vi "SLL DE DAQ Parameters LV2 Global.vi"(6 "Option":T6, 8 "Error in (no error)":errorcluster, 11 "Global Info":T1={"Enable Engines"={"AI Enable"=TRUE, "AO Enable"=TRUE, "DI Enable"=TRUE, "DO Enable"=TRUE}, "DAQ Control Type"={"Analog Input"=enum."Finite", "Analog Output"=enum."Finite", "Digital Input"=enum."Finite", "Digital Output"=enum."Finite"}, "DAQ Parameters"={"AI Sampling Rate (Samples/Sec)"=1000.0, "MvgAVG Window Size (# of Points)"=1000, "Enable Filter"=TRUE, "Enable MvgAVG"=TRUE, "Circular Buffer Size (Sec)"=1000.0, "AO Sampling Rate (Samples/Sec)"=1000.0, "Graph Update Rate (Samples/Sec)"=0.0, "File Logging Rate (Samples/Sec)"=500}, "AO Safe Values"=[], "DO Safe Values"=[], "DO Interconnected Lines"=[], "AI Channels Unit"=[], "Units Information"=[]}) -> (0 "Error out":errorcluster, 3 "Global Info":T1={"Enable Engines"={"AI Enable"=TRUE, "AO Enable"=TRUE, "DI Enable"=TRUE, "DO Enable"=TRUE}, "DAQ Control Type"={"Analog Input"=enum."Finite", "Analog Output"=enum."Finite", "Digital Input"=enum."Finite", "Digital Output"=enum."Finite"}, "DAQ Parameters"={"AI Sampling Rate (Samples/Sec)"=1000.0, "MvgAVG Window Size (# of Points)"=1000, "Enable Filter"=TRUE, "Enable MvgAVG"=TRUE, "Circular Buffer Size (Sec)"=1000.0, "AO Sampling Rate (Samples/Sec)"=1000.0, "Graph Update Rate (Samples/Sec)"=0.0, "File Logging Rate (Samples/Sec)"=500}, "AO Safe Values"=[], "DO Safe Values"=[], "DO Interconnected Lines"=[], "AI Channels Unit"=[], "Units Information"=[]})   [LabVIEW 2013]
uses:
  Sub VIs/DAQ Engine/Controls/SLL DE DAQ Parameters LV2Global Options.ctl
  Sub VIs/DAQ Engine/Controls/SLL DE DAQ Engine Parameters.ctl
  Sub VIs/DAQ Engine/Controls/SLL DE List of Analog Outputs.ctl
  Sub VIs/DAQ Engine/Controls/SLL DE List of Digital Outputs.ctl
  Sub VIs/DAQ Engine/Controls/SLL DE List of Analog Inputs.ctl
  Sub VIs/DAQ Engine/Controls/SLL DE List of AI Channel Type.ctl
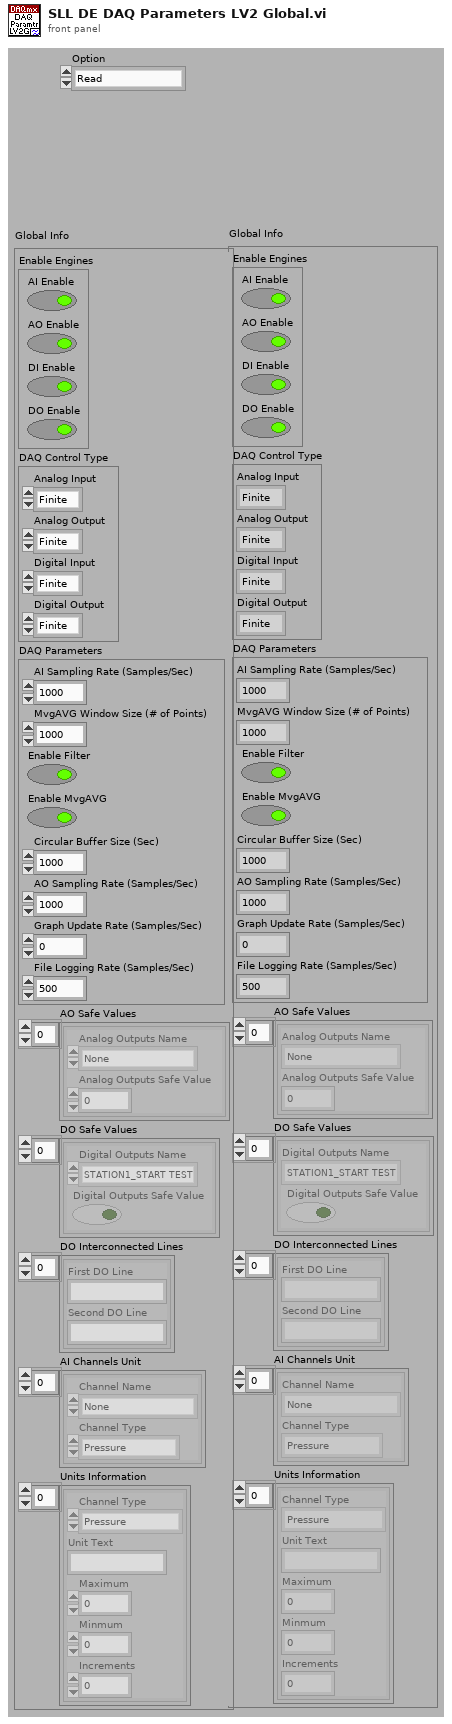
[diagram p1: front panel]
types:
  T1 = typedef "SLL DE DAQ Engine Parameters.ctl" = cluster{"Enable Engines":cluster{"AI Enable":bool, "AO Enable":bool, "DI Enable":bool, "DO Enable":bool}, "DAQ Control Type":cluster{"Analog Input":enum16{"Finite", "Continuous", "Driver"}, "Analog Output":enum16{"Finite", "Continuous", "Driver"}, "Digital Input":enum16{"Finite", "Continuous", "Driver"}, "Digital Output":enum16{"Finite", "Continuous", "Driver"}}, "DAQ Parameters":cluster{"AI Sampling Rate (Samples/Sec)":dbl, "MvgAVG Window Size (# of Points)":i32, "Enable Filter":bool, "Enable MvgAVG":bool, "Circular Buffer Size (Sec)":dbl, "AO Sampling Rate (Samples/Sec)":dbl, "Graph Update Rate (Samples/Sec)":dbl, "File Logging Rate (Samples/Sec)":i32}, "AO Safe Values":cluster{"Analog Outputs Name":T2, "Analog Outputs Safe Value":dbl}[], "DO Safe Values":cluster{"Digital Outputs Name":T3, "Digital Outputs Safe Value":bool}[], "DO Interconnected Lines":cluster{"First DO Line":string, "Second DO Line":string}[], "AI Channels Unit":cluster{"Channel Name":T4, "Channel Type":T5}[], "Units Information":cluster{"Channel Type":T5, "Unit Text":string, "Maximum":dbl, "Minmum":dbl, "Increments":dbl}[]}
  T2 = typedef "SLL DE List of Analog Outputs.ctl" = enum16{"None"}
  T3 = typedef "SLL DE List of Digital Outputs.ctl" = enum16{"STATION1_START TEST", "STATION1_STOP TEST", "STATION1_LIGHT1", "STATION1_LIGHT2", "STATION1_LIGHT3", "STATION1_SELECT_TEST", "STATION2_START TEST", "STATION2_STOP TEST", "STATION2_LIGHT1", "STATION2_LIGHT2", "STATION2_LIGHT3", "STATION2_SELECT_TEST", "STATION3_START TEST", "STATION3_STOP TEST", "STATION3_LIGHT1", "STATION3_LIGHT2", "STATION3_LIGHT3", "STATION3_SELECT_TEST", "STATION4_START TEST", "STATION4_STOP TEST", "STATION4_LIGHT1", "STATION4_LIGHT2", "STATION4_LIGHT3", "STATION4_SELECT_TEST"}
  T4 = typedef "SLL DE List of Analog Inputs.ctl" = enum16{"None"}
  T5 = typedef "SLL DE List of AI Channel Type.ctl" = enum16{"Pressure", "Flow", "Temperature", "Time Scale", "Voltage", "Current", "Frequency", "Sound", "Speed", "Torque", "Distance", "Channel Type 1", "Channel Type 2", "Channel Type 3"}
  T6 = typedef "SLL DE DAQ Parameters LV2Global Options.ctl" = enum16{"Read", "Write"}
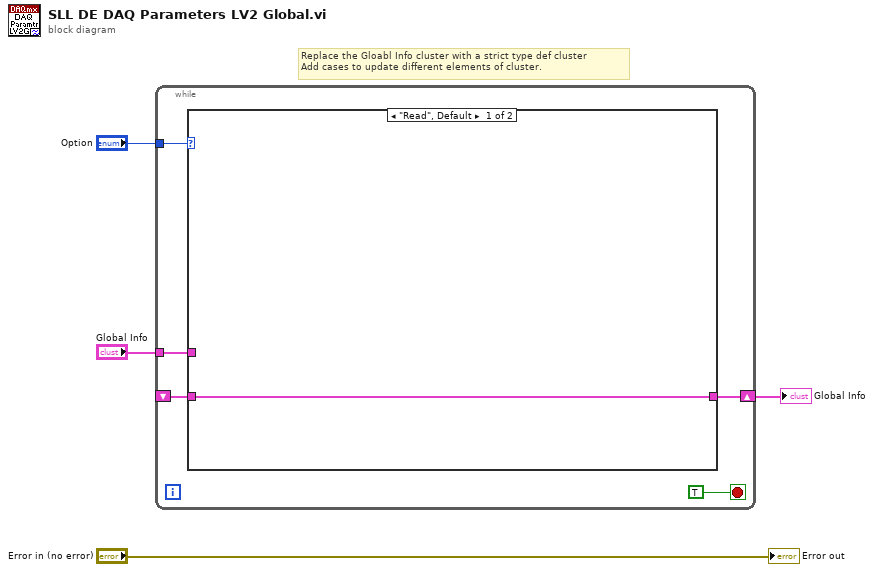
[diagram p0: block diagram]
diagram:
  # "Replace the Gloabl Info cluster with a strict type def cluster\nAdd cases to update different elements of cluster."
  n1 = while {
    tunnel: "Option" -> [w8]
    shift-right: [w7] -> w2
    shift-left: _ -> [w6]
    tunnel: "Global Info" -> [w5]
    stop <- TRUE stop-if-true
    n2 = case shown="\"Read\", Default" w8 {
      tunnel: [w10 w11] -> w7
      tunnel: w6 -> [w10 _]
      tunnel: w5 -> [_ w11]
      frame "Read", Default {
      }
      frame "Write" {
      }
    }
  }
  "Global Info" <- w2
  "Error out" <- "Error in (no error)"
